vi "SetZeroFCG.vi"(8 "error in (no error)":errorcluster) -> (0 "error out":errorcluster)   [LabVIEW 2013]
uses:
  Variables/ccdChipPixels.vi
  Variables/GlobalSetGetConfigureCamera.vi
  Variables/GlobalSetGetHeidenhainParameters.vi
  Variables/GlobalSetNumberOfDigits_PhysikalInstruments.vi
  Variables/GlobalGetMesaurementStatus.vi
  Variables/GlobalExitVar.vi
  Variables/GrapRoi.vi
  Variables/GlobalGetPhysikalInstrumentsOnOff.vi
  Variables/StartStopMesaurement.vi
  Variables/GlobalLaserEmissionOnOffInterlook.vi
  Variables/GlobalGetHeidenhainDriftOnOff.vi
  Variables/GlobalGetConfigurationStatus.vi
  Variables/GlobalGetInitialisationStatus.vi
  Variables/GlobalGetKoherasLaserOnOff.vi
  Variables/GlobalGetAOTFOnOff.vi
  Variables/GlobalGetAvantesSpectrometerOnOff.vi
  Variables/GlobalGetCamerasOnOff.vi
  Variables/SetRoi.vi
  Variables/GetPicture.vi
  Variables/StopGetPic.vi
  Variables/GlobalSetGetParametersAvantes.vi
  Variables/GlobalSetGetPixelOfRoi.vi
  Variables/GetSetGlobalPath2StoreStackData.vi
  Variables/GlobalCameraDebugTemperature.vi
  Variables/ScannerMirrorStatus.vi
  Variables/GlobalGetSetMeasurementType.vi
  Variables/GlobalSetNumberOfDigits_Scanners.vi
  Variables/AOTF_NonLinearLinesOnOff.vi
  Variables/GlobalImage.vi
  Variables/GlobalGetBeamDiagnostics.vi
  Variables/GlobalStopGetBeamDiagnostics.vi
panel:
  in  "out":T1
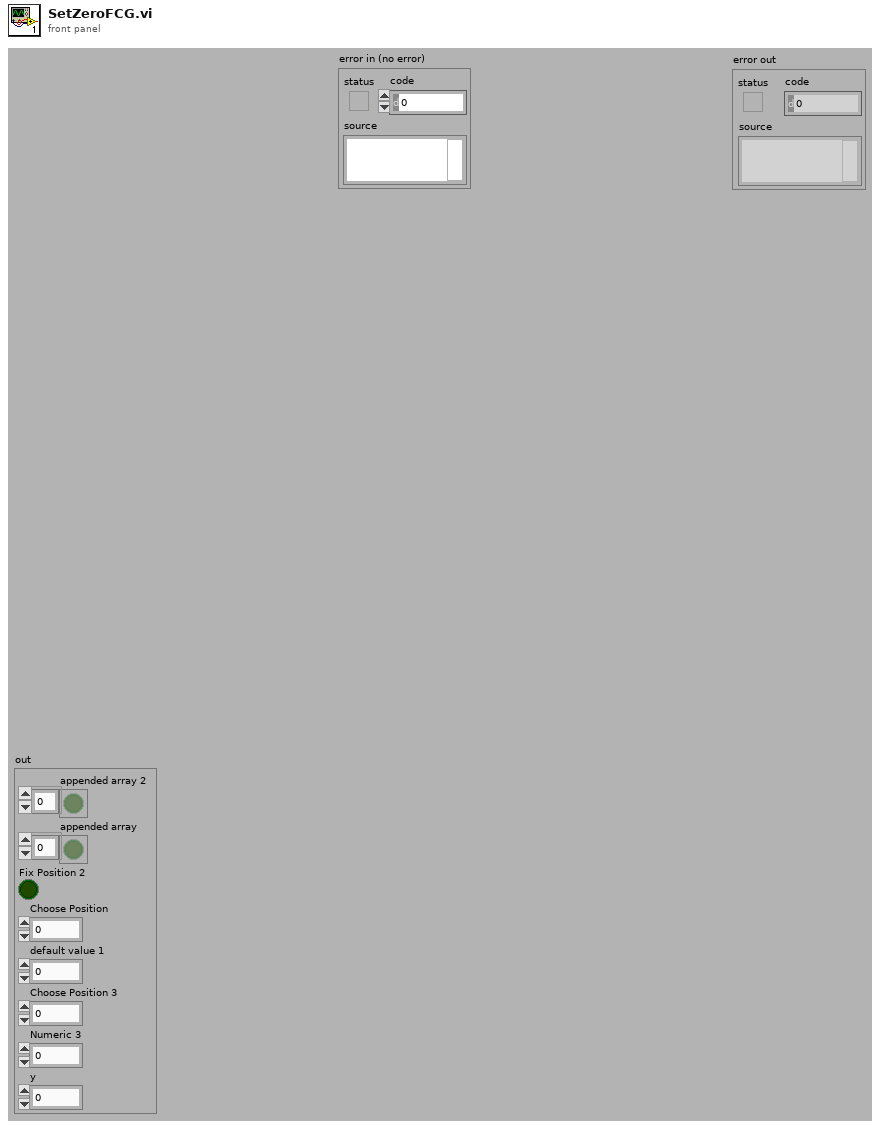
[diagram p1: front panel]
types:
  T1 = cluster{"appended array 2":bool[], "appended array":bool[], "Fix Position 2":bool, "Choose Position":dbl, "default value 1":dbl, "Choose Position 3":dbl, "Numeric 3":i32, "y":i32}
  T2 = cluster{"numbers of \nmeasurements":i16, "startPixel":u16, "stopPixel":u16, "intTime / [ms]":sgl, "backgroundSubtract":bool, "numAvg":u32}
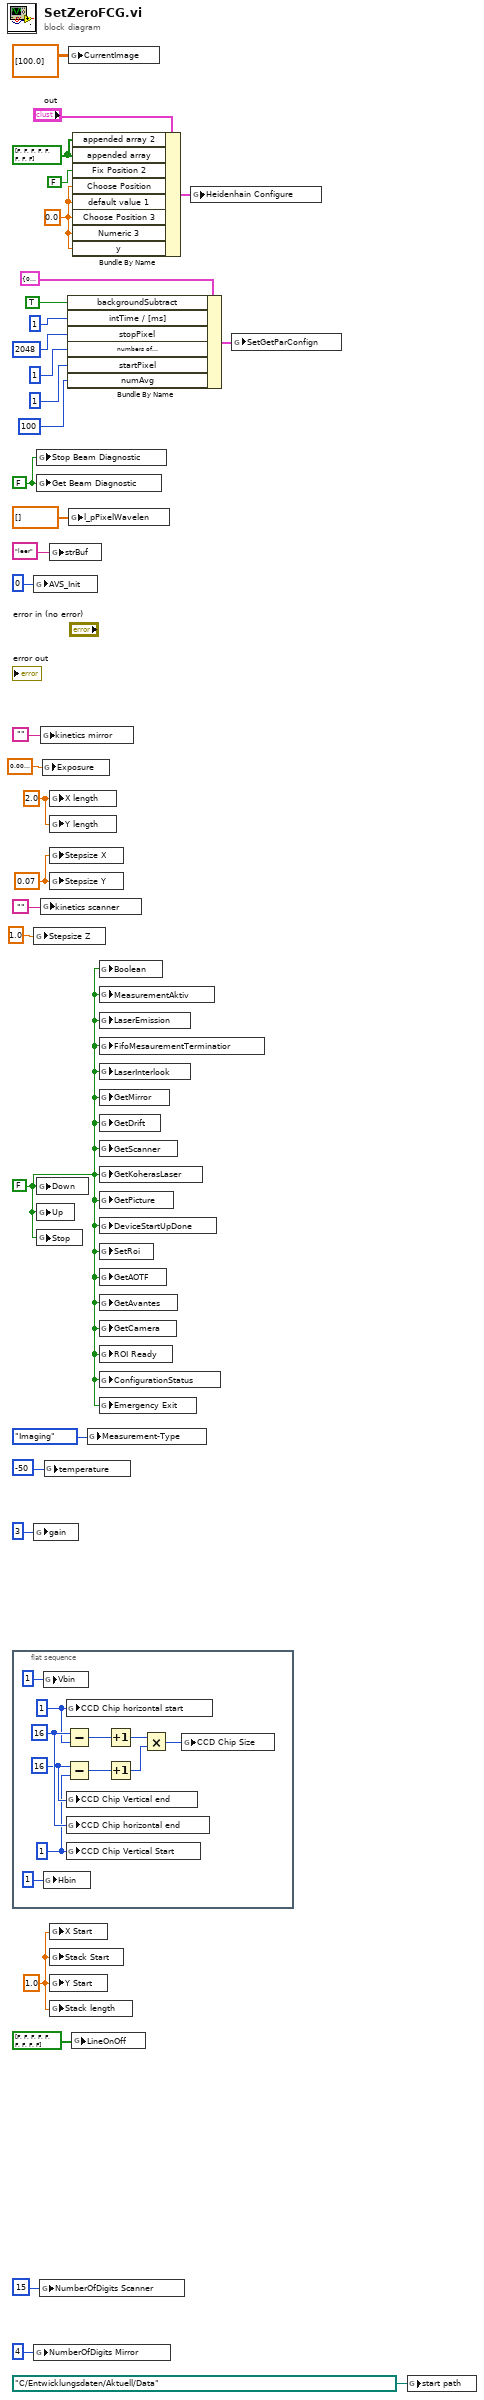
[diagram p0: block diagram]
diagram:
  w3 = FALSE ("Stop Beam Diagnostic")
  w12 = 2.0 ("X length")
  w15 = 1.0 ("X Start")
  w13 = 0.07 ("Pixel SizeX")
  w2 = FALSE ("andor 2")
  w31 = 0.0 ("Choose Position")
  w32 = bool[] [FALSE, FALSE, FALSE, FALSE, FALSE, FALSE, FALSE, FALSE] ("appended array")
  n1 = flat-sequence {
    frame #0 {
      w37 = 16 ("CCD Chip Vertical end")
      w34 = 1 ("CCD Chip Vertical Start")
      w36 = 16 ("CCD Chip horizontal end")
      w35 = 1
      n2 = global write "GlobalSetGetConfigureCamera.vi" "Vbin"(1 ("Vbin")) -> ()
      n3 = global write "GlobalSetGetConfigureCamera.vi" "Hbin"(1 ("Hbin")) -> ()
      n4 = Subtract(x=w37, y=w35) -> (x-y=w39:i32)
      n5 = Subtract(x=w36, y=w34) -> (x-y=w38:i32)
      n6 = global write "ccdChipPixels.vi" "CCD Chip horizontal start"(w35) -> ()
      n7 = global write "ccdChipPixels.vi" "CCD Chip Vertical end"(w36) -> ()
      n8 = global write "ccdChipPixels.vi" "CCD Chip horizontal end"(w37) -> ()
      n9 = global write "ccdChipPixels.vi" "CCD Chip Vertical Start"(w34) -> ()
      n10 = Increment(x=w39) -> (x+1=w41:i32)
      n11 = Increment(x=w38) -> (x+1=w40:i32)
      n12 = Multiply(x=w41, y=w40) -> (x*y=w44:i32)
      n13 = global write "ccdChipPixels.vi" "CCD Chip Size"(w44) -> ()
    }
  }
  n14 = global write "GlobalSetGetParametersAvantes.vi" "AVS_Init"(0 ("AVS_Init")) -> ()
  n15 = global write "GlobalSetGetPixelOfRoi.vi" "Stepsize Z"(1.0 ("Stepsize Z")) -> ()
  n16 = global write "GlobalSetGetConfigureCamera.vi" "gain"(3 ("gain")) -> ()
  n17 = global write "GlobalSetNumberOfDigits_PhysikalInstruments.vi" "NumberOfDigits Mirror"(4 ("NumberOfDigits")) -> ()
  n18 = global write "GlobalStopGetBeamDiagnostics.vi" "Stop Beam Diagnostic"(w3) -> ()
  n19 = global write "GlobalGetBeamDiagnostics.vi" "Get Beam Diagnostic"(w3) -> ()
  n20 = global write "GlobalSetGetHeidenhainParameters.vi" "Down"(w2) -> ()
  n21 = global write "GlobalSetGetHeidenhainParameters.vi" "Up"(w2) -> ()
  n22 = global write "StopGetPic.vi" "Stop"(w2) -> ()
  n23 = global write "GlobalSetNumberOfDigits_Scanners.vi" "NumberOfDigits Scanner"(15 ("NumberOfDigits Scanner")) -> ()
  n24 = global write "ScannerMirrorStatus.vi" "kinetics mirror"("") -> ()
  n25 = global write "ScannerMirrorStatus.vi" "kinetics scanner"("") -> ()
  n26 = global write "GlobalSetGetConfigureCamera.vi" "Exposure"(sgl 0.01 ("ExpTime")) -> ()
  n27 = global write "GlobalCameraDebugTemperature.vi" "temperature"(-50 ("temperature")) -> ()
  n28 = global write "GlobalSetGetParametersAvantes.vi" "strBuf"("leer" ("strBuf")) -> ()
  n29 = global write "GlobalSetGetPixelOfRoi.vi" "X length"(w12) -> ()
  n30 = global write "GlobalSetGetPixelOfRoi.vi" "Y length"(w12) -> ()
  n31 = global write "GlobalSetGetPixelOfRoi.vi" "Stepsize X"(w13) -> ()
  n32 = global write "GlobalSetGetPixelOfRoi.vi" "Stepsize Y"(w13) -> ()
  n33 = global write "GlobalSetGetPixelOfRoi.vi" "X Start"(w15) -> ()
  n34 = global write "GlobalSetGetPixelOfRoi.vi" "Stack Start"(w15) -> ()
  n35 = global write "GlobalSetGetPixelOfRoi.vi" "Y Start"(w15) -> ()
  n36 = global write "GlobalSetGetPixelOfRoi.vi" "Stack length"(w15) -> ()
  n37 = Bundle By Name(cluster=T2 {"numbers of \nmeasurements"=0, "startPixel"=0, "stopPixel"=0, "intTime / [ms]"=0.0, "backgroundSubtract"=FALSE, "numAvg"=0} ("out"), "backgroundSubtract"=TRUE, "intTime / [ms]"=u16 1 ("startPixel"), "stopPixel"=u16 2048, "numbers of \nmeasurements"=i16 1 ("numbers of \nmeasurements"), "startPixel"=u16 1, "numAvg"=u32 100) -> (w20:T2)
  n38 = global write "GlobalImage.vi" "CurrentImage"(dbl[][] [[100.0]] ("CurrentImage")) -> ()
  n39 = global write "GlobalSetGetParametersAvantes.vi" "l_pPixelWavelen"(dbl[] [] ("l_pPixelWavelen")) -> ()
  n40 = global write "AOTF_NonLinearLinesOnOff.vi" "LineOnOff"(bool[] [FALSE, FALSE, FALSE, FALSE, FALSE, FALSE, FALSE, FALSE, FALSE] ("LineOnOff")) -> ()
  n41 = Bundle By Name(cluster="out", "appended array 2"=w32, "appended array"=w32, "Fix Position 2"=FALSE, "Choose Position"=w31, "default value 1"=w31, "Choose Position 3"=w31, "Numeric 3"=w31, "y"=w31) -> (w21:T1)
  n42 = global write "GlobalGetSetMeasurementType.vi" "Measurement-Type"(enum32{"Diffusion", "Imaging"}."Imaging" ("Measurement-Type")) -> ()
  n43 = global write "StartStopMesaurement.vi" "Boolean"(w2) -> ()
  n44 = global write "GlobalGetMesaurementStatus.vi" "MeasurementAktiv"(w2) -> ()
  n45 = global write "GlobalLaserEmissionOnOffInterlook.vi" "LaserEmission"(w2) -> ()
  n46 = global write "GlobalGetMesaurementStatus.vi" "FifoMesaurementTerminatior"(w2) -> ()
  n47 = global write "GlobalLaserEmissionOnOffInterlook.vi" "LaserInterlook"(w2) -> ()
  n48 = global write "GlobalGetPhysikalInstrumentsOnOff.vi" "GetMirror"(w2) -> ()
  n49 = global write "GlobalGetHeidenhainDriftOnOff.vi" "GetDrift"(w2) -> ()
  n50 = global write "GlobalGetPhysikalInstrumentsOnOff.vi" "GetScanner"(w2) -> ()
  n51 = global write "GlobalGetKoherasLaserOnOff.vi" "GetKoherasLaser"(w2) -> ()
  n52 = global write "GetPicture.vi" "GetPicture"(w2) -> ()
  n53 = global write "GlobalGetInitialisationStatus.vi" "DeviceStartUpDone"(w2) -> ()
  n54 = global write "SetRoi.vi" "SetRoi"(w2) -> ()
  n55 = global write "GlobalGetAOTFOnOff.vi" "GetAOTF"(w2) -> ()
  n56 = global write "GlobalGetAvantesSpectrometerOnOff.vi" "GetAvantes"(w2) -> ()
  n57 = global write "GlobalGetCamerasOnOff.vi" "GetCamera"(w2) -> ()
  n58 = global write "GrapRoi.vi" "ROI Ready"(w2) -> ()
  n59 = global write "GlobalGetConfigurationStatus.vi" "ConfigurationStatus"(w2) -> ()
  n60 = global write "GlobalExitVar.vi" "Emergency Exit"(w2) -> ()
  n61 = global write "GlobalSetGetHeidenhainParameters.vi" "Heidenhain Configure"(w21) -> ()
  n62 = global write "GlobalSetGetParametersAvantes.vi" "SetGetParConfign"(w20) -> ()
  n63 = global write "GetSetGlobalPath2StoreStackData.vi" "start path"(path "C:/Entwicklungsdaten/Aktuell/Data" ("start path")) -> ()
